vi "DST800 Com.vi"() -> ()   [LabVIEW 2016, in "DST800.lvlib"]
uses:
  DST800.lvlib
  <vilib>/Instr/_visa.llb/VISA Configure Serial Port (Instr).vi
panel:
  out "depth":cluster{"时间标识":timestamp, "深度":dbl}
  in  "启动":bool
  out "匹配字段":string
  in  "停止":bool
  out "字符串":string
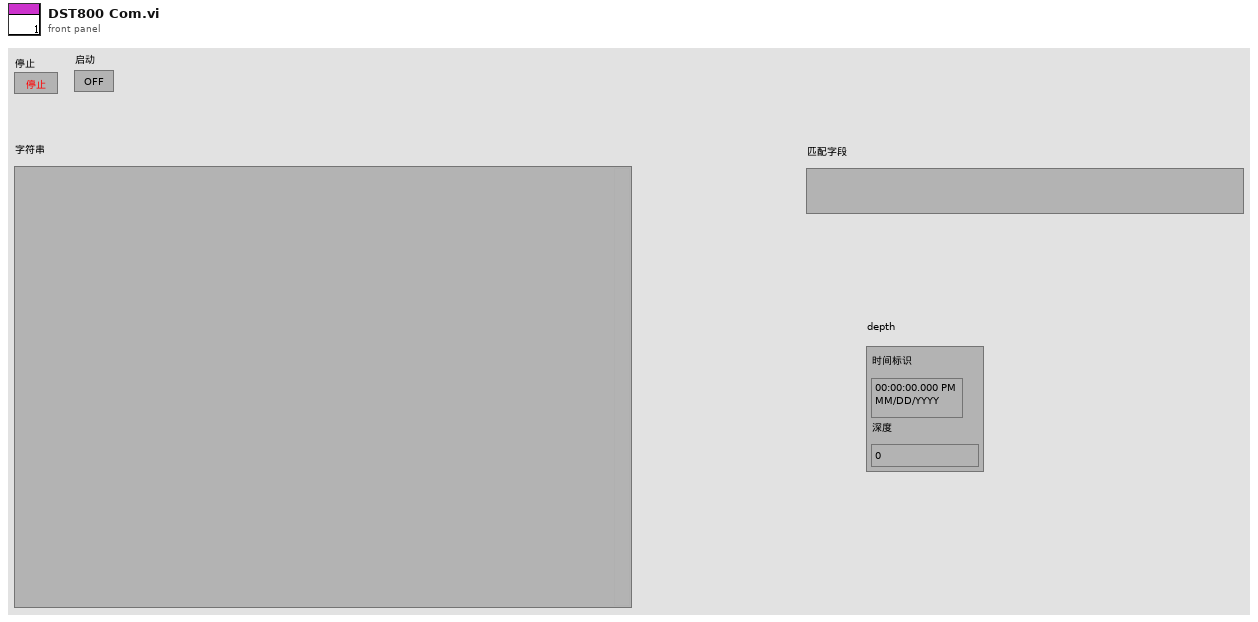
[diagram p1: front panel]
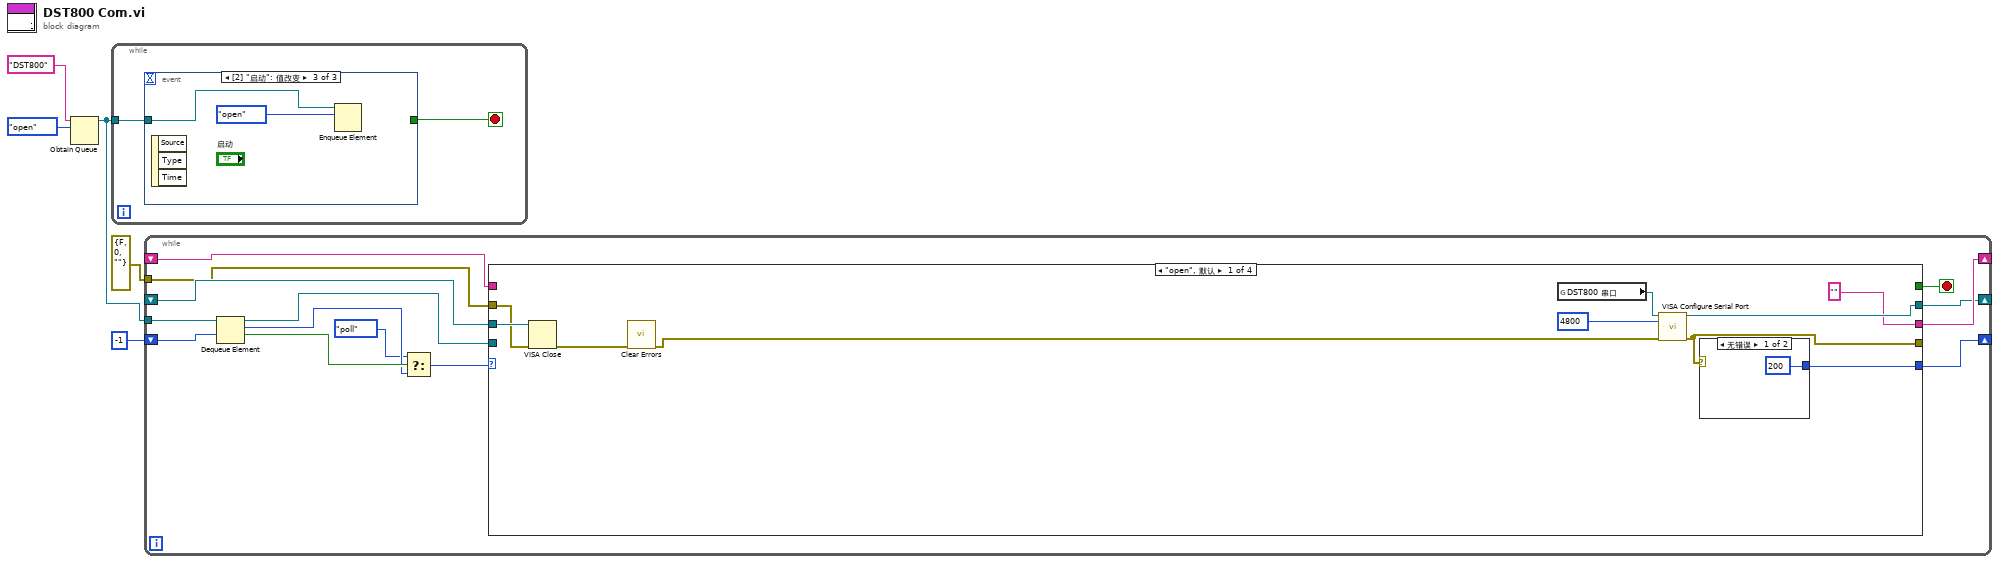
[diagram p0: block diagram]
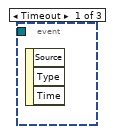
[diagram p2: hidden frame]
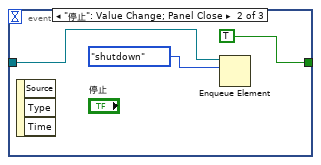
[diagram p3: hidden frame]
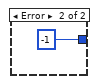
[diagram p4: hidden frame]
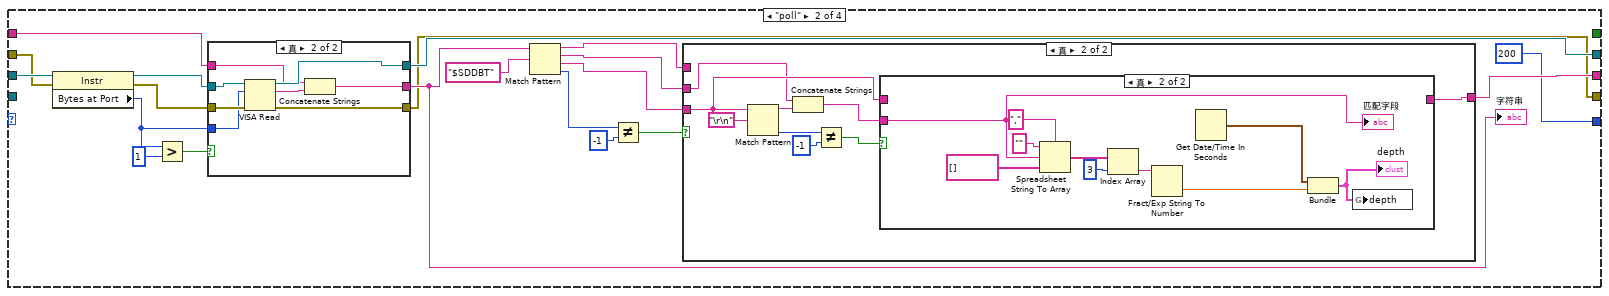
[diagram p5: hidden frame]
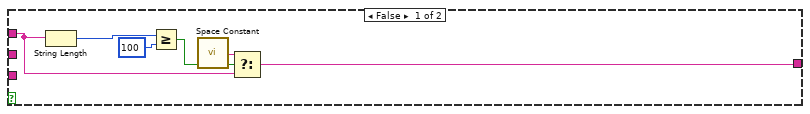
[diagram p6: hidden frame]
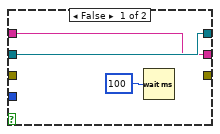
[diagram p8: hidden frame]
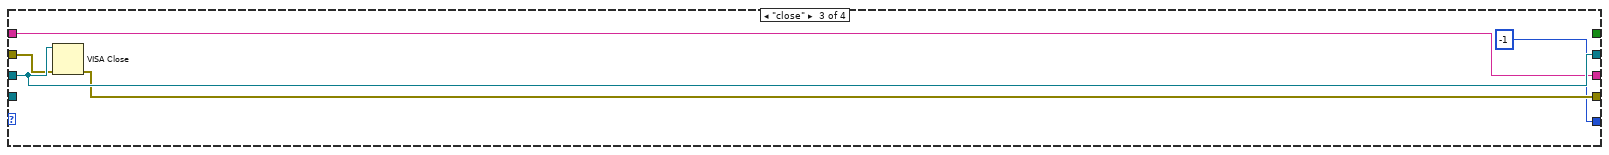
[diagram p9: hidden frame]
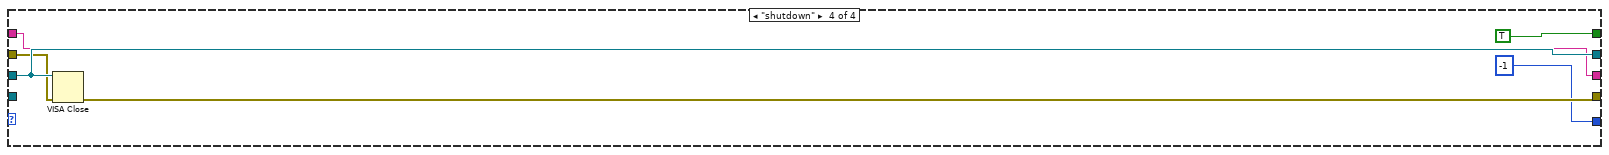
[diagram p10: hidden frame]
diagram:
  n1 = Obtain Queue(name (unnamed)="DST800" ("名称（未命名）"), element data type=enum16{"open", "poll", "close", "shutdown"}."open" ("枚举")) -> (queue out=w3:refnum<queue>)  [unwired: 3 in, 2 out]
  n2 = while {
    tunnel: w3 -> [w6]
    stop <- w7 stop-if-true
    n3 = event shown="[2] \"启动\": 值改变" {
      selector: _ -> [_ _ _]
      dyn-events: _ -> [_ _ _]
      timeout: _ -> [_ _ _]
      tunnel: [_ TRUE _] -> w7
      tunnel: w6 -> [_ w9 w12]
      event Timeout {
        n4 = event-data() -> ()  [unwired: 1 in, 3 out]
      }
      event "停止": Value Change; Panel Close {
        n5 = event-data() -> ()  [unwired: 1 in, 3 out]
        n6 = Enqueue Element(queue=w9, element=enum16{"open", "poll", "close", "shutdown"}."shutdown" ("元素")) -> ()  [unwired: 2 in, 3 out]
      }
      event "启动": Value Change {
        n7 = event-data() -> ()  [unwired: 1 in, 3 out]
        n8 = Enqueue Element(queue=w12, element=enum16{"open", "poll", "close", "shutdown"}."open" ("元素")) -> ()  [unwired: 2 in, 3 out]
      }
    }
  }
  n9 = while {
    tunnel: w3 -> [w26]
    shift-right: [w13] -> _
    shift-left: _ -> [w24]
    shift-right: [w23] -> _
    shift-left: _ -> [w22]
    tunnel: errorcluster {"status"=FALSE, "code"=0, "source"=""} ("错误输入（无错误）") -> [w20]
    shift-right: [w18] -> _
    shift-left: -1 ("超时毫秒(-1)") -> [w19]
    stop <- w21 stop-if-true
    n10 = Dequeue Element(queue=w26, timeout in ms (-1)=w19) -> (queue out=w25:refnum<queue>, element=w16:enum16{"open", "poll", "close", "shutdown"}, timed out?=w17:bool)  [unwired: 1 in, 1 out]
    n11 = Select(t=enum16{"open", "poll", "close", "shutdown"}."poll", s=w17, f=w16) -> (s? t:f=w15:enum16{"open", "poll", "close", "shutdown"})
    n12 = case shown="\"open\", 默认" w15 {
      tunnel: w25 -> [_ _ _ _]
      tunnel: [w35 w46 w100 w106] -> w13
      tunnel: w24 -> [w34 w47 w100 w106]
      tunnel: ["" ("String") w45 w99 w104] -> w23
      tunnel: w22 -> [_ w44 w99 w104]
      tunnel: [_ _ _ TRUE] -> w21
      tunnel: w20 -> [w32 w42 w98 w103]
      tunnel: [w31 w43 w97 w102] -> _
      tunnel: [w30 200 ("超时毫秒(-1)") -1 ("超时毫秒(-1)") -1 ("超时毫秒(-1)")] -> w18
      frame "open", Default {
        n13 = VISA Close(VISA resource name=w34, error in (no error)=w32) -> (error out=w29:errorcluster)
        n14 = call <vilib>:"Clear Errors.vi"("error in (no error)"=w29) -> ("error out"=w28:errorcluster)  [unwired: 5 in, 1 out]
        n15 = global read "DST800全局变量.vi" "DST800 串口"() -> (w27:refnum<visa-resource-name>)
        n16 = call-poly "VISA Configure Serial Port"("VISA resource name"=w27, "baud rate (9600)"=u32 4800, "error in (no error)"=w28) -> ("VISA resource name out"=w35:refnum<visa-resource-name>, "error out"=w31:errorcluster)  [unwired: 11 in]
        n17 = case shown="无错误" w31 {
          tunnel: [200 ("超时毫秒(-1)") -1 ("超时毫秒(-1)")] -> w30
          frame No Error {
          }
          frame Error {
          }
        }
      }
      frame "poll" {
        n18 = property class="Instr"(reference=w47, error in=w42) -> (reference out=w49:refnum<visa-resource-name>, error out=w50:errorcluster, "Bytes at Port"=w40:u32)
        n19 = Greater?(x=w40, y=u32 1) -> (0:w48:bool)
        n20 = case shown="真" w48 {
          tunnel: w49 -> [w87 w95]
          tunnel: w50 -> [_ w94]
          tunnel: [w87 w93] -> w46
          tunnel: [_ w92] -> w43
          tunnel: [w85 w89] -> w56
          tunnel: w44 -> [w85 w91]
          tunnel: w40 -> [_ w88]
          frame False {
            n21 = Wait (ms)(milliseconds to wait=u32 100 ("等待时间（毫秒）")) -> ()  [unwired: 1 out]
          }
          frame True {
            n22 = VISA Read(VISA resource name=w95, byte count=w88, error in (no error)=w94) -> (VISA resource name out=w93:refnum<visa-resource-name>, read buffer=w90:string, error out=w92:errorcluster)  [unwired: 1 out]
            n23 = Concatenate Strings(w91, w90) -> (w89:string)
          }
        }
        "字符串" <- w56
        n24 = Match Pattern(string=w56, regular expression="$SDDBT" ("正则表达式")) -> (before substring=w58:string, match substring=w57:string, after substring=w52:string, offset past match=w53:i32)  [unwired: 1 in]
        n25 = Not Equal?(x=w53, y=-1) -> (x != y?=w55:bool)
        n26 = case shown="真" w55 {
          tunnel: w52 -> [_ w70]
          tunnel: [w61 w69] -> w45
          tunnel: w57 -> [_ w67]
          tunnel: w58 -> [w59 _]
          frame False {
            n27 = String Length(string=w59) -> (length=w64:i32)
            n28 = Greater Or Equal?(x=w64, y=100) -> (x >= y?=w62:bool)
            n29 = call <vilib>:"Space Constant.vi"() -> ("String"=w60:string)
            n30 = Select(t=w60, s=w62, f=w59) -> (s? t:f=w61:string)
          }
          frame True {
            n31 = Match Pattern(string=w70, regular expression="\r\n") -> (before substring=w66:string, offset past match=w73:i32)  [unwired: 1 in, 2 out]
            n32 = Concatenate Strings(w67, w66) -> (w65:string)
            n33 = Not Equal?(x=w73, y=-1) -> (x != y?=w71:bool)
            n34 = case shown="真" w71 {
              tunnel: w65 -> [_ w82]
              tunnel: [w74 _] -> w69
              tunnel: w70 -> [w74 _]
              frame False {
              }
              frame True {
                n35 = Spreadsheet String To Array(delimiter (Tab)="," ("分隔符(Tab)"), format string="" ("格式字符串"), spreadsheet string=w82, array type (2D Dbl)=string[] []) -> (array=w80:string[])
                n36 = Index Array(array=w80, index=3 ("索引")) -> (element=w78:string)
                n37 = Fract/Exp String To Number(string=w78) -> (number=w76:dbl)  [unwired: 3 in, 1 out]
                n38 = Get Date/Time In Seconds() -> (seconds since 1Jan1904=w77:timestamp)
                n39 = Bundle("seconds since 1Jan1904"=w77, w76) -> (w75:cluster{"seconds since 1Jan1904":timestamp, dbl})  [unwired: 1 in]
                "depth" <- w75
                n40 = global write "DST800全局变量.vi" "depth"(w75) -> ()
                "匹配字段" <- w82
              }
            }
          }
        }
      }
      frame "close" {
        n41 = VISA Close(VISA resource name=w100, error in (no error)=w98) -> (error out=w97:errorcluster)
      }
      frame "shutdown" {
        n42 = VISA Close(VISA resource name=w106, error in (no error)=w103) -> (error out=w102:errorcluster)
      }
    }
  }
